vi "Publish Packages to Package Repositoryvi.vi"(7 "String in":refnum<vi>, 8 "error in (no error)":errorcluster, 9 "Repository Name":string, 10 "vip paths":path[](array[path])) -> (0 "error out":errorcluster, 1 "Repository Folder Location":path, 2 "Package Names Published":string[](array[string]))   [LabVIEW 2019, in "Build.lvlib"]
uses:
  Build.lvlib
  <vilib>/JKI/VIPM API/VIPM API_vipm_api.lvlib
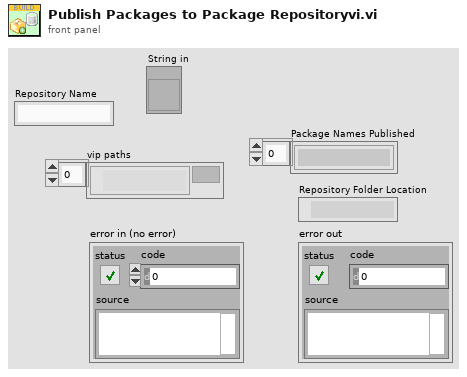
[diagram p1: front panel]
types:
  T1 = typedef "VIPM API_vipm_api.lvlib/Repository Info Cluster_vipm_api.ctl" = cluster{"Repository Name":string, "Repository Folder Location":path}
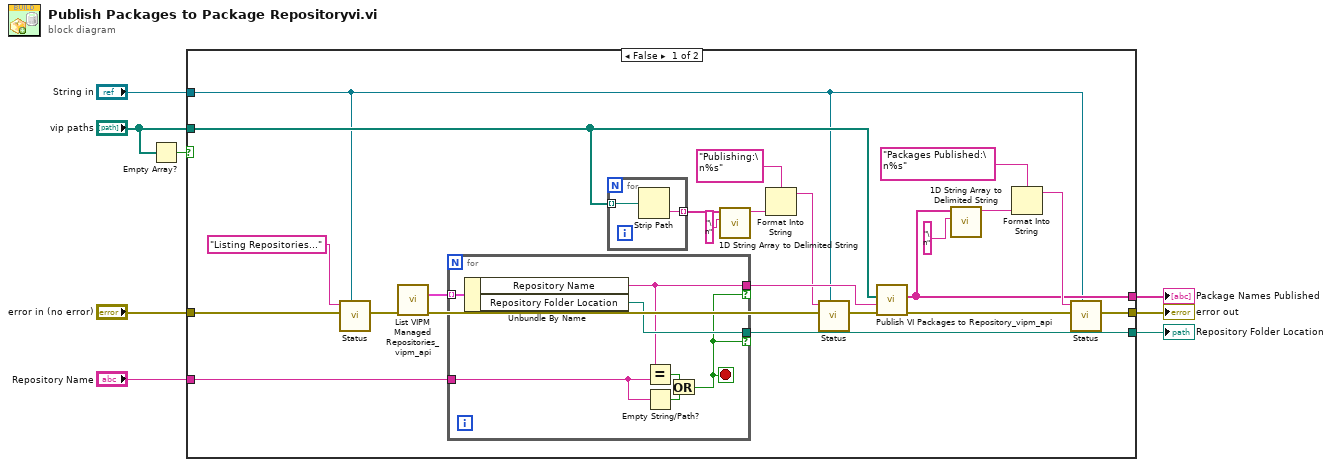
[diagram p0: block diagram]
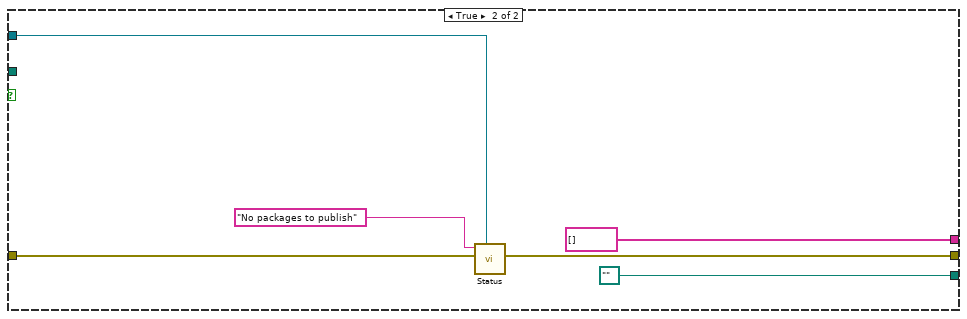
[diagram p2: hidden frame]
diagram:
  n1 = Empty Array?(array="vip paths") -> (empty?=w3:bool)
  n2 = case shown="False" w3 {
    tunnel: [w9 path "" ("Repository Folder Location")] -> w8
    tunnel: [w30 w44] -> w7
    tunnel: "vip paths" -> [w20 _]
    tunnel: [w15 string[] [] ("Package Names Published")] -> w6
    tunnel: "error in (no error)" -> [w14 w46]
    tunnel: "String in" -> [w12 w45]
    tunnel: "Repository Name" -> [w10 _]
    frame False {
      n3 = call "Status.vi"("Status Indicator Reference"=w12, "error in (no error)"=w14, "Status"="Listing Repositories..." ("format string")) -> ("error out"=w13:errorcluster)  [unwired: 8 in]
      n4 = call <vilib>:"List VIPM Managed Repositories_vipm_api.vi"("error in (no error)"=w13) -> ("Managed Repositories Info"=w16:T1[], "error out"=w19:errorcluster)  [unwired: 13 in]
      n5 = for {
        tunnel: [w36] -> w25 if=w33
        tunnel: w16 -> [w38] mode=indexing
        tunnel: [w37] -> w9 if=w33
        tunnel: w10 -> [w32]
        stop <- w33 stop-if-true
        n6 = Unbundle By Name(w38) -> ("Repository Name"=w36:string, "Repository Folder Location"=w37:path)
        n7 = Equal?(x=w36, y=w32) -> (x = y?=w34:bool)
        n8 = Empty String/Path?(string/path=w32) -> (empty?=w35:bool)
        n9 = Or(x=w34, y=w35) -> (x .or. y?=w33:bool)
      }
      n10 = for {
        tunnel: w20 -> [w40] mode=indexing
        tunnel: [w39] -> w28 mode=indexing
        n11 = Strip Path(path=w40) -> (name=w39:string)  [unwired: 1 out]
      }
      n12 = call <vilib>:"1D String Array to Delimited String.vi"("delimiter"="\n", "string array"=w28) -> ("delimited string"=w22:string)  [unwired: 9 in]
      n13 = Format Into String(format string="Publishing:\n%s", w22) -> (resulting string=w24:string)  [unwired: 2 in, 1 out]
      n14 = call "Status.vi"("Status Indicator Reference"=w12, "error in (no error)"=w19, "Status"=w24) -> ("error out"=w18:errorcluster)  [unwired: 8 in]
      n15 = call <vilib>:"Publish VI Packages to Repository_vipm_api.vi"("error in (no error)"=w18, "Repository Name"=w25, "Packages to publish to Repository Library (vip,ogp)"=w20) -> ("error out"=w26:errorcluster, "Package Names Published"=w15:string[])  [unwired: 7 in]
      n16 = call <vilib>:"1D String Array to Delimited String.vi"("delimiter"="\n", "string array"=w15) -> ("delimited string"=w31:string)  [unwired: 9 in]
      n17 = Format Into String(format string="Packages Published:\n%s", w31) -> (resulting string=w29:string)  [unwired: 2 in, 1 out]
      n18 = call "Status.vi"("Status Indicator Reference"=w12, "error in (no error)"=w26, "Status"=w29) -> ("error out"=w30:errorcluster)  [unwired: 8 in]
    }
    frame True {
      n19 = call "Status.vi"("Status Indicator Reference"=w45, "error in (no error)"=w46, "Status"="No packages to publish" ("format string")) -> ("error out"=w44:errorcluster)  [unwired: 8 in]
    }
  }
  "Repository Folder Location" <- w8
  "Package Names Published" <- w6
  "error out" <- w7
